vi "Remove.vi"(0 "object in":refnum<class "Tree.lvclass">, 5 "Error In":errorcluster) -> (14 "object out":refnum<class "Tree.lvclass">, 19 "Error Out":errorcluster)   [LabVIEW 2024, in "Tree.lvclass"]
uses:
  <resource>/Framework/Providers/Open_GDS/ClassProviders/Provider_LvNativeClass/Templates/NativeBaseTemplate/NativeBaseTemplate.lvclass/NativeBaseTemplate.ctl
  Tree.lvclass
  Tree.lvclass/Tree.ctl
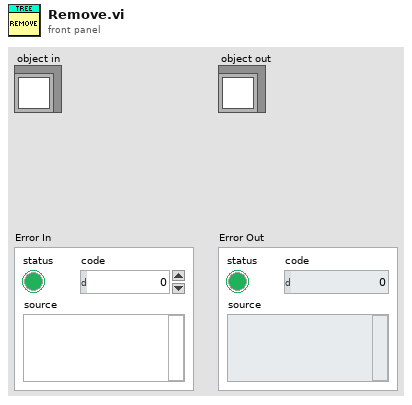
[diagram p1: front panel]
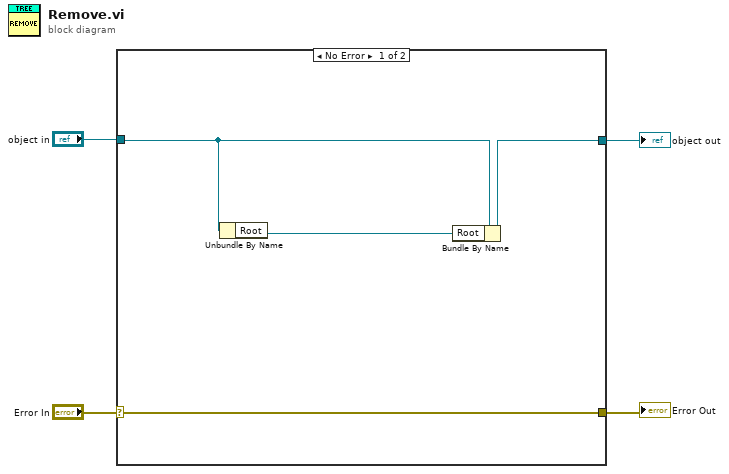
[diagram p0: block diagram]
diagram:
  n1 = case shown="No Error" "Error In" {
    selector: "Error In" -> [w7 w10]
    tunnel: [w7 w10] -> w3
    tunnel: [w5 w9] -> w1
    tunnel: "object in" -> [w6 w9]
    frame No Error {
      n2 = Unbundle By Name(w6) -> ("Root"=w8:refnum<class "Node.lvclass">)
      n3 = Bundle By Name(cluster=w6, "Root"=w8) -> (w5:refnum<class "Tree.lvclass">)
    }
    frame Error {
    }
  }
  "Error Out" <- w3
  "object out" <- w1
